vi "JSON Command Seperation Test.vi"() -> ()   [LabVIEW 2021]
uses:
  <vilib>/regexp/Match Regular Expression.xnode
  TCP Engine/TCP Engine.lvlib
  <userlib>/_OpenG.lib/string/string.llb/openg_string.lvlib
panel:
  out "Array":string[](array[string])
  out "number":i32
  out "lines":string[](array[string])
  out "Data":string
  out "SubCmd":string
  out "Command":string
  out "Interface":string
  in  "JSON String":string
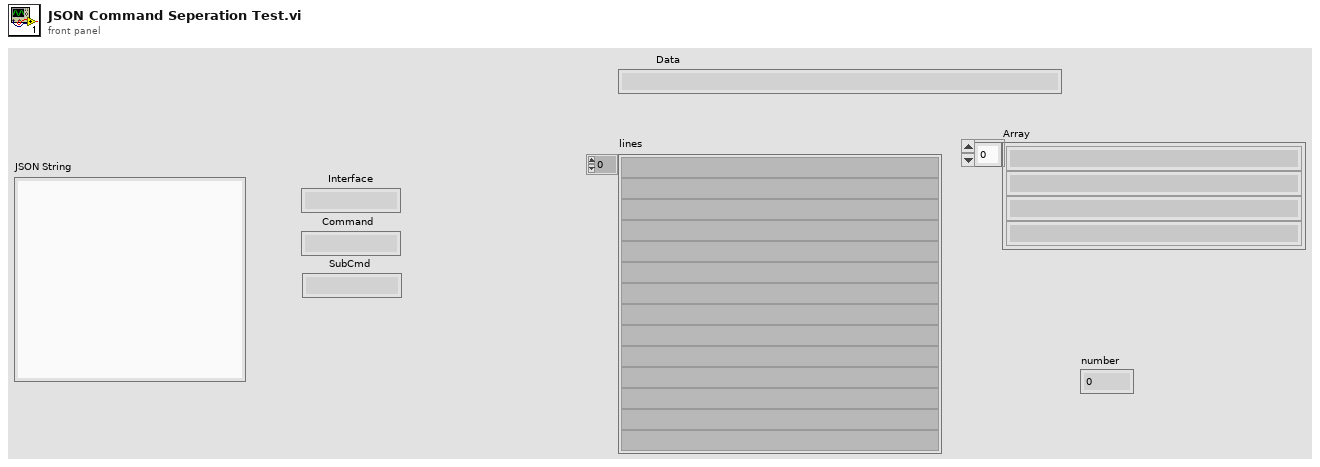
[diagram p1: front panel]
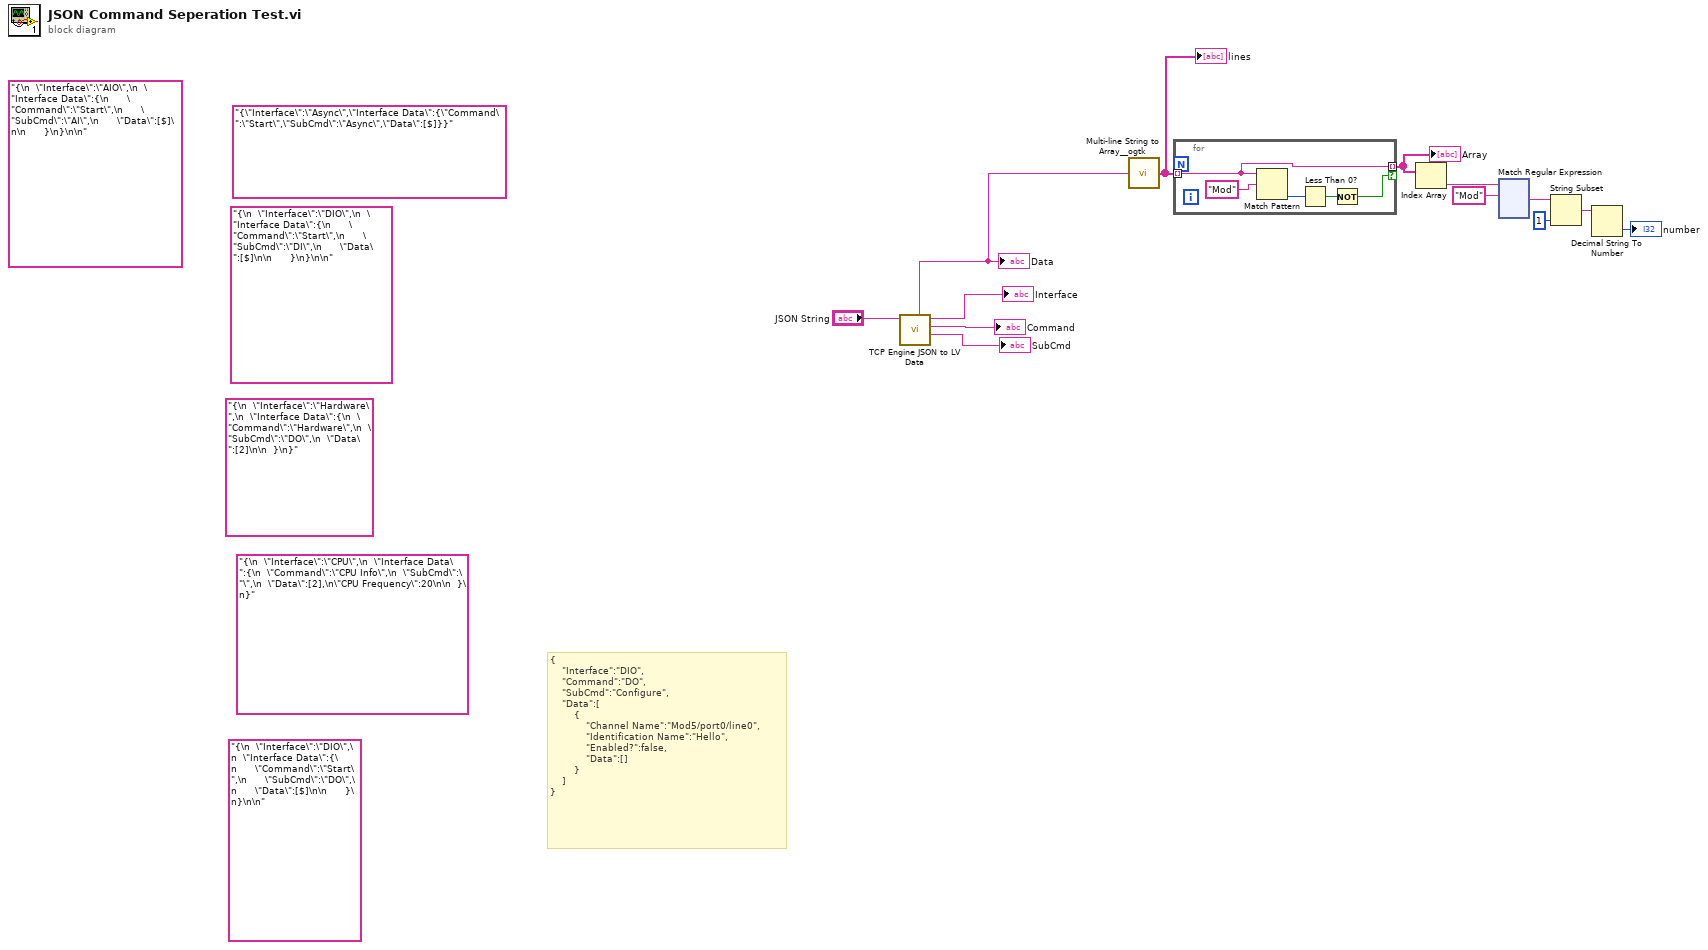
[diagram p0: block diagram]
diagram:
  (unwired) "{\n  \"Interface\":\"DIO\",\n  \"Interface Data\":{\n      \"Command\":\"Start\",\n      \"SubCmd\":\"DO\",\n      \"Data\":[$]\n\n      }\n}\n\n" ("AI_start")
  (unwired) "{\n  \"Interface\":\"DIO\",\n  \"Interface Data\":{\n      \"Command\":\"Start\",\n      \"SubCmd\":\"DI\",\n      \"Data\":[$]\n\n      }\n}\n\n" ("AI_start")
  (unwired) "{\n  \"Interface\":\"AIO\",\n  \"Interface Data\":{\n      \"Command\":\"Start\",\n      \"SubCmd\":\"AI\",\n      \"Data\":[$]\n\n      }\n}\n\n" ("AI_start")
  (unwired) "{\n  \"Interface\":\"CPU\",\n  \"Interface Data\":{\n  \"Command\":\"CPU Info\",\n  \"SubCmd\":\"\",\n  \"Data\":[2],\n\"CPU Frequency\":20\n\n  }\n}" ("Data 2")
  (unwired) "{\n  \"Interface\":\"Hardware\",\n  \"Interface Data\":{\n  \"Command\":\"Hardware\",\n  \"SubCmd\":\"DO\",\n  \"Data\":[2]\n\n  }\n}" ("Data 2")
  (unwired) "{\"Interface\":\"Async\",\"Interface Data\":{\"Command\":\"Start\",\"SubCmd\":\"Async\",\"Data\":[$]}}" ("AI_start")
  # "{\n    \"Interface\":\"DIO\",\n    \"Command\":\"DO\",\n    \"SubCmd\":\"Configure\",\n    \"Data\":[\n        {\n            \"Channel Name\":\"Mod5/port0/line0\",\n            \"Identification Name\":\"Hello\",\n            \"Enabled?\":false,\n            \"Data\":[]\n        }\n    ]\n}"
  n1 = call "TCP Engine JSON to LV Data.vi"("JSON String"="JSON String") -> ("SubCmd"=→"SubCmd":string, "Command"=→"Command":string, "Interface"=→"Interface":string, "Data"=w9:string)  [unwired: 5 in, 2 out]
  "Data" <- w9
  n2 = call <userlib>:"Multi-line String to Array__ogtk.vi"("string"=w9) -> ("lines"=w2:string[])
  "lines" <- w2
  n3 = for {
    tunnel: w2 -> [w14] mode=indexing
    tunnel: [w14] -> w1 mode=indexing if=w15
    n4 = Match Pattern(string=w14, regular expression="Mod") -> (offset past match=w17:i32)  [unwired: 1 in, 3 out]
    n5 = Less Than 0?(x=w17) -> (x < 0?=w16:bool)
    n6 = Not(x=w16) -> (.not. x?=w15:bool)
  }
  "Array" <- w1
  n7 = Index Array(array=w1) -> (element=w7:string)  [unwired: 1 in]
  n8 = xnode "Match Regular Expression"("input string"=w7, "regular expression"="Mod") -> ("after match"=w6:string)  [unwired: 4 in, 4 out]
  n9 = String Subset(string=w6, length (rest)=1 ("length (rest)")) -> (substring=w4:string)  [unwired: 1 in]
  n10 = Decimal String To Number(string=w4) -> (number=→"number":i32)  [unwired: 2 in, 1 out]
